vi "8XY5.vi"(11 "Variables and Memory in":T1 {"GFX" format="%02x"}) -> (3 "Variables and Memory out":T1 {"GFX" format="%02x"})   [LabVIEW 2021]
uses:
  Controls/ClusterF.ctl
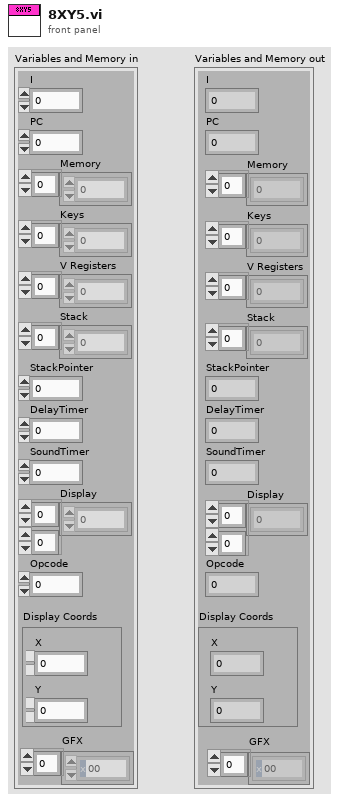
[diagram p1: front panel]
types:
  T1 = typedef "ClusterF.ctl" = cluster{"I":u16, "PC":u16, "Memory":u8[], "Keys":u8[], "V Registers":u8[], "Stack":u16[], "StackPointer":u16, "DelayTimer":u8, "SoundTimer":u8, "Display":u8[][], "Opcode":u16, "Display Coords":cluster{"X":u8, "Y":u8}, "GFX":u8[]}
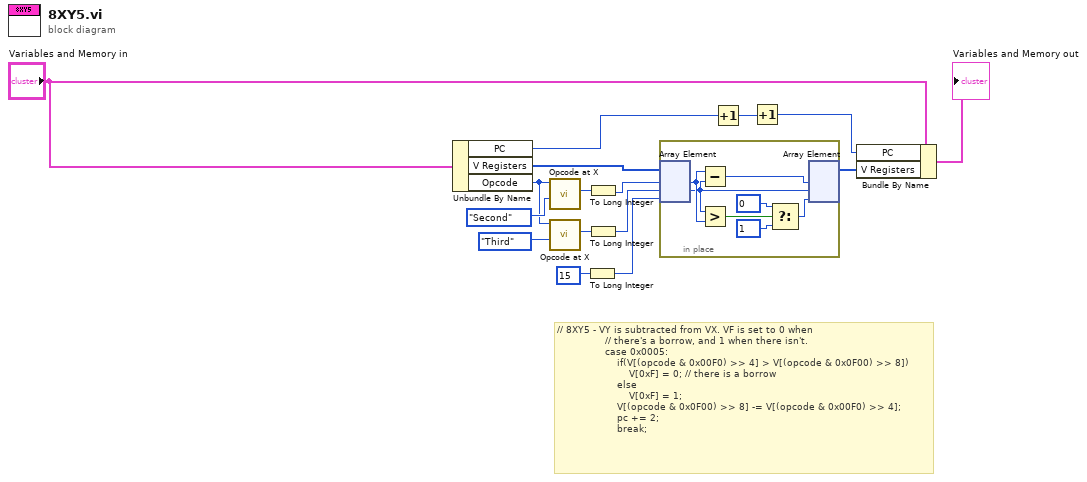
[diagram p0: block diagram]
diagram:
  # "// 8XY5 - VY is subtracted from VX. VF is set to 0 when\n                // there's a borrow, and 1 when there isn't.\n                case 0x0005:\n                    if(V[(opcode & 0x00F0) >> 4] > V[(opcode & 0x0F00) >> 8])\n                        V[0xF] = 0; // there is a borrow\n                    else\n                        V[0xF] = 1;\n                    V[(opcode & 0x0F00) >> 8] -= V[(opcode & 0x00F0) >> 4];\n                    pc += 2;\n                    break;"
  n1 = Unbundle By Name("Variables and Memory in") -> ("PC"=w1:u16, "V Registers"=w11:u8[], "Opcode"=w4:u16)
  n2 = call "Opcode at X.vi"("X Position"=enum16{"First", "Second", "Third", "Fourth"}."Second", "Opcode"=w4) -> ("Opcode at X Position (U8)"=w8:u8)  [unwired: 9 in]
  n3 = call "Opcode at X.vi"("X Position"=enum16{"First", "Second", "Third", "Fourth"}."Third", "Opcode"=w4) -> ("Opcode at X Position (U8)"=w7:u8)  [unwired: 9 in]
  n4 = To Long Integer(number=15) -> (32bit integer=w16:i32)
  n5 = To Long Integer(number=w8) -> (32bit integer=w12:i32)
  n6 = To Long Integer(number=w7) -> (32bit integer=w15:i32)
  n7 = in-place {
    n8 = in-place-array #1(w11, w12, w15, w16) -> (w22:u8, w17:u8)  [unwired: 1 out]
    n9 = Subtract(x=w22, y=w17) -> (x-y=w23:u8)
    n10 = Greater?(x=w17, y=w22) -> (0:w21:bool)
    n11 = Select(t=u8 0, s=w21, f=u8 1) -> (s? t:f=w18:u8)
    n12 = in-place-array #1(w23, w17, w18) -> (w14:u8[])  [unwired: 3 out]
  }
  n13 = Increment(x=w1) -> (x+1=w2:u16)
  n14 = Increment(x=w2) -> (x+1=w3:u16)
  n15 = Bundle By Name(cluster="Variables and Memory in", "PC"=w3, "V Registers"=w14) -> (→"Variables and Memory out":T1)
